vi "Set DAQNodes Dict.vi"(8 "error in (no error)":errorcluster, 10 "DAQ Node Dict DVR":T1, 11 "DAQ":refnum<class "DAQ.lvclass">) -> (0 "error out":errorcluster, 3 "DAQ":refnum<class "DAQ.lvclass">)   [LabVIEW 2017, in "DAQ.lvclass"]
doc: "Developed by Kevin Thompson\nkevin@thompsonengineering.net\n\nCopyright 2018-2020\nThompson Engineering, LLC"
uses:
  DAQ.lvclass
  <vilib>/TELLC/Dynamic CVT API/TD Dynamic CVT DVR--ref.ctl
  DAQ.lvclass/DAQ.ctl
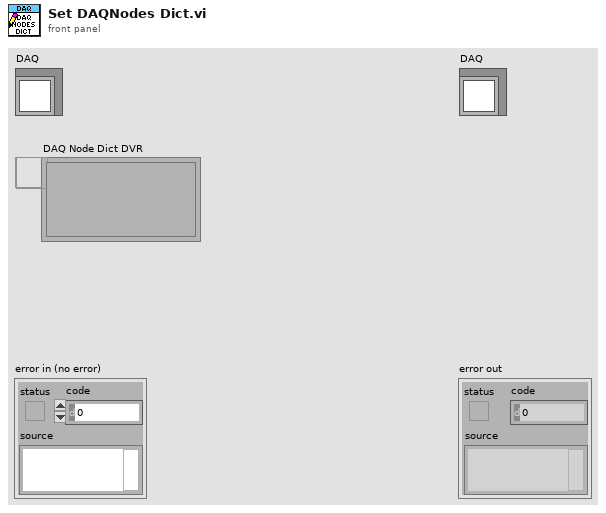
[diagram p1: front panel]
types:
  T1 = typedef "TD Dynamic CVT DVR--ref.ctl" = refnum<data-value>
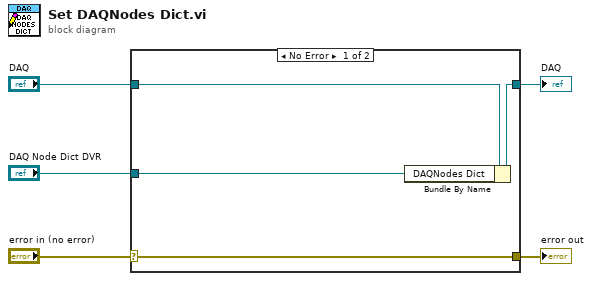
[diagram p0: block diagram]
diagram:
  n1 = case shown="No Error" "error in (no error)" {
    selector: "error in (no error)" -> [w9 w10]
    tunnel: [w9 w10] -> w4
    tunnel: [w7 w11] -> w2
    tunnel: "DAQ" -> [w8 w11]
    tunnel: "DAQ Node Dict DVR" -> [w6 _]
    frame No Error {
      n2 = Bundle By Name(cluster=w8, "DAQNodes Dict"=w6) -> (w7:refnum<class "DAQ.lvclass">)
    }
    frame Error {
    }
  }
  "error out" <- w4
  "DAQ" <- w2
